vi "xy.vi"(11 "Array":dbl[][](array[numeric])) -> (3 "xy":cluster{"Array":dbl[], "Array":dbl[]})   [LabVIEW 2013]
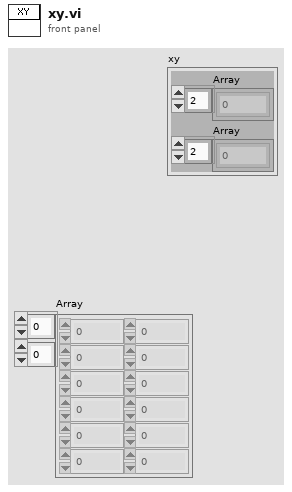
[diagram p1: front panel]
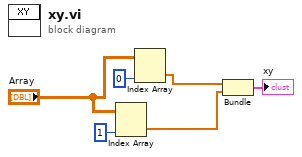
[diagram p0: block diagram]
diagram:
  n1 = Index Array(array="Array", index (col)=1 ("disabled index (col)")) -> (element=w2:dbl[])  [unwired: 1 in]
  n2 = Index Array(array="Array", index (col)=0 ("disabled index (col)")) -> (element=w3:dbl[])  [unwired: 1 in]
  n3 = Bundle("Array"=w3, "Array"=w2) -> (→"xy":cluster{"Array":dbl[], "Array":dbl[]})  [unwired: 1 in]
